vi "Tree Test.vi"() -> ()   [LabVIEW 2023]
uses:
  Glyph .NET Drawer/Drawer .Net.lvclass
  E:/Labview/LV 2023/Libs/LV Symbol/Font Glyph Drawer Interface/Glyph Drawer/Glyph Drawer.lvclass
  Font Glyph Drawer Interface/Tree Control Canvas/Tree Control Canvas.lvclass
  E:/Labview/LV 2023/Libs/LV Symbol/Font Glyph Drawer Interface/Glyph Canvas/Glyph Canvas.lvclass
  LV-Awesome/LV Awesome/LV Awesome.lvclass
  E:/Labview/LV 2023/Libs/LV Symbol/Font Glyph Drawer Interface/Glyph Source/Glyph Source.lvclass
  Font Glyph Drawer Interface/Transform/Transform.lvclass
  Font Glyph Drawer Interface/Glyph Canvas/Glyph Canvas.lvclass
panel:
  in  "Tree":string(tree)
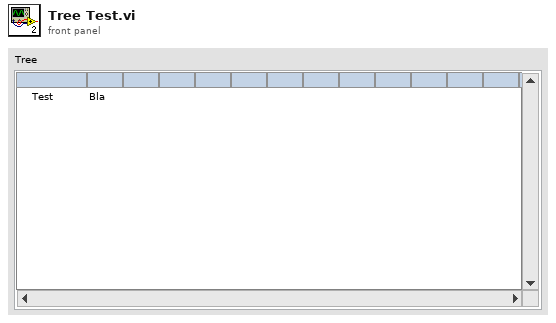
[diagram p1: front panel]
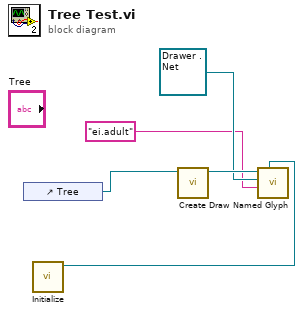
[diagram p0: block diagram]
diagram:
  n1 = control-ref of="Tree"() -> (w5:refnum<vi>)
  n2 = call "Initialize.vi"() -> ("LV Awesome"=w2:refnum<class "LV Awesome.lvclass">)  [unwired: 10 in, 1 out]
  n3 = call "Create.vi"("Tree"=w5) -> ("Picture Control Canvas out"=w4:refnum<class "Tree Control Canvas.lvclass">)  [unwired: 9 in, 1 out]
  n4 = call "Draw Named Glyph.vi"("Glyph Source in"=w2, "Glyph Name"="ei.adult", "Glyph Drawer in"=refnum<class "Drawer .Net.lvclass"> refnum ("Glyph .NET.lvlib:Drawer .Net.lvclass"), "Glyph Canvas in"=w4) -> ()  [unwired: 5 in, 3 out]
